vi "Find Path.vi"(8 "error in (no error)":errorcluster, 9 "channel 2":string, 10 "channel 1":string, 11 "SLSC Switch in":refnum<class "SLSC Switch.lvclass">) -> (0 "error out":errorcluster, 2 "Relay Indexes":i32[](array[numeric]), 3 "SLSC Switch out":refnum<class "SLSC Switch.lvclass">)   [LabVIEW 2016, in "SLSC Switch.lvlib" / "SLSC Switch.lvclass"]
uses:
  SLSC Switch.lvclass
  SLSC Switch.lvclass/SLSC Switch.ctl
  Relay/Relay.lvclass/Relay.ctl
  Relay/Read relay name.vi
  Switch Action Processor/Switch Action Processor.lvclass
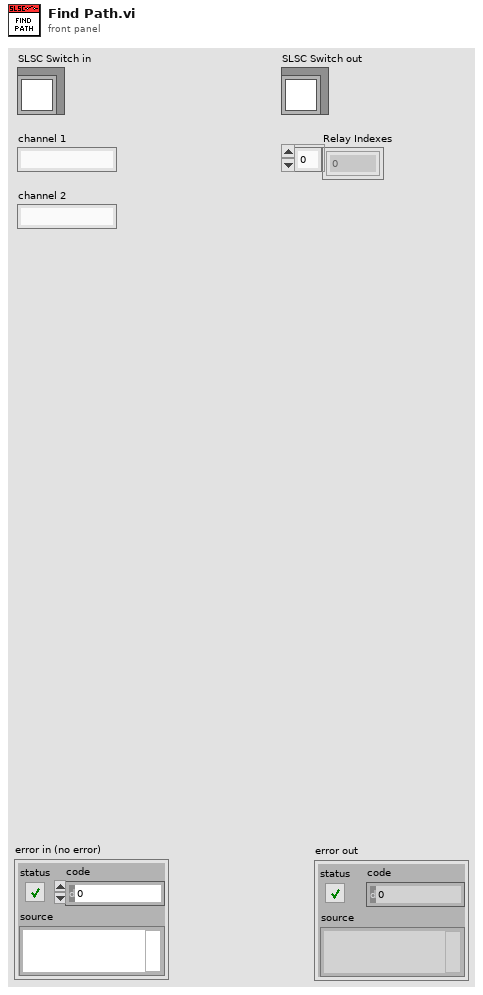
[diagram p1: front panel]
types:
  T1 = typedef "SLSC Switch.lvlib/SLSC Switch.lvclass/Topology.ctl" = cluster{"name":string, "InitialState":T2, "ChannelList":T3, "ConnectionList":T4[], "MuxList":cluster{"Src":string, "Dests":string[]}[]}
  T2 = typedef "SLSC Switch.lvlib/SLSC Switch.lvclass/JSON.InitialState.ctl" = cluster{"Open":string[], "Close":string[]}
  T3 = typedef "SLSC Switch.lvlib/SLSC Switch.lvclass/JSON.ChannelList.ctl" = cluster{"Names":string[]}
  T4 = typedef "SLSC Switch.lvlib/SLSC Switch.lvclass/JSON.ConnectionList.ctl" = cluster{"Src":string, "Dest":string, "Relays":string[]}
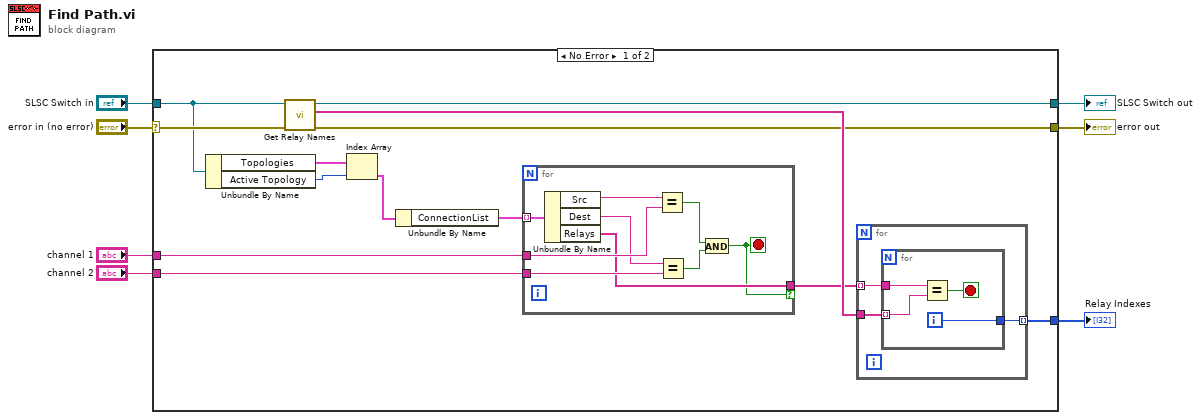
[diagram p0: block diagram]
diagram:
  n1 = case shown="No Error" "error in (no error)" {
    selector: "error in (no error)" -> [w14 w37]
    tunnel: [w20 _] -> w7
    tunnel: [w18 w38] -> w6
    tunnel: "SLSC Switch in" -> [w11 w38]
    tunnel: "channel 2" -> [w16 _]
    tunnel: "channel 1" -> [w15 _]
    tunnel: [w13 w37] -> w1
    frame No Error {
      n2 = Unbundle By Name(w11) -> ("Topologies"=w10:T1[], "Active Topology"=w12:i32)
      n3 = call "Get Relay Names.vi"("error in (no error)"=w14, "SLSC Switch in"=w11) -> ("error out"=w13:errorcluster, "Relay Names"=w19:string[], "SLSC Switch out"=w18:refnum<class "SLSC Switch.lvclass">)  [unwired: 7 in]
      n4 = Index Array(array=w10, index=w12) -> (element=w8:T1)
      n5 = Unbundle By Name(w8) -> ("ConnectionList"=w9:T4[])
      n6 = for {
        tunnel: w9 -> [w29] mode=indexing
        tunnel: w15 -> [w27]
        tunnel: w16 -> [w25]
        tunnel: [w22] -> w17 if=w21
        stop <- w21 stop-if-true
        n7 = Unbundle By Name(w29) -> ("Src"=w28:string, "Dest"=w26:string, "Relays"=w22:string[])
        n8 = Equal?(x=w28, y=w27) -> (x = y?=w24:bool)
        n9 = Equal?(x=w26, y=w25) -> (x = y?=w23:bool)
        n10 = And(x=w24, y=w23) -> (x .and. y?=w21:bool)
      }
      n11 = for {
        tunnel: w17 -> [w31] mode=indexing
        tunnel: w19 -> [w32]
        tunnel: [w30] -> w20 mode=indexing
        n12 = for {
          tunnel: w32 -> [w36] mode=indexing
          tunnel: w31 -> [w35]
          tunnel: [w33] -> w30
          i -> [w33]
          stop <- w34 stop-if-true
          n13 = Equal?(x=w35, y=w36) -> (x = y?=w34:bool)
        }
      }
    }
    frame Error {
    }
  }
  "Relay Indexes" <- w7
  "SLSC Switch out" <- w6
  "error out" <- w1
